vi "Parse Response JSON.vi"(8 "error in (no error)":errorcluster, 10 "Response JSON":string, 11 "RGetSceneList in":refnum<class "RGetSceneList.lvclass">) -> (0 "error out":errorcluster, 3 "RGetSceneList out":refnum<class "RGetSceneList.lvclass">)   [LabVIEW 2022 SP3, in "obs-websocket-lv.lvlib" / "RGetSceneList.lvclass"]
uses:
  RGetSceneList.lvclass
  RGetSceneList.lvclass/RGetSceneList.ctl
  <vilib>/IlluminatedG/lv-web-crypto/lv-json/JSON/JSON.lvlib
  Scene.ctl
  obs-websocket-lv.lvlib
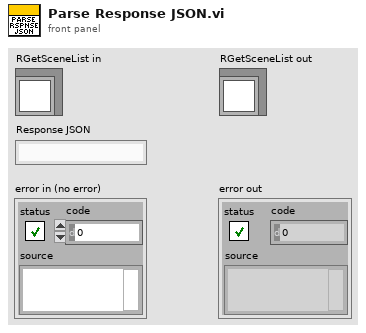
[diagram p1: front panel]
types:
  T1 = typedef "JSON.lvlib/JSON Item Type.ctl" = enum16{"unknown", "null", "Array", "Object", "String", "Number", "Boolean"}
  T2 = typedef "obs-websocket-lv.lvlib/Scene.ctl" = cluster{"Index":i32, "Name":string}
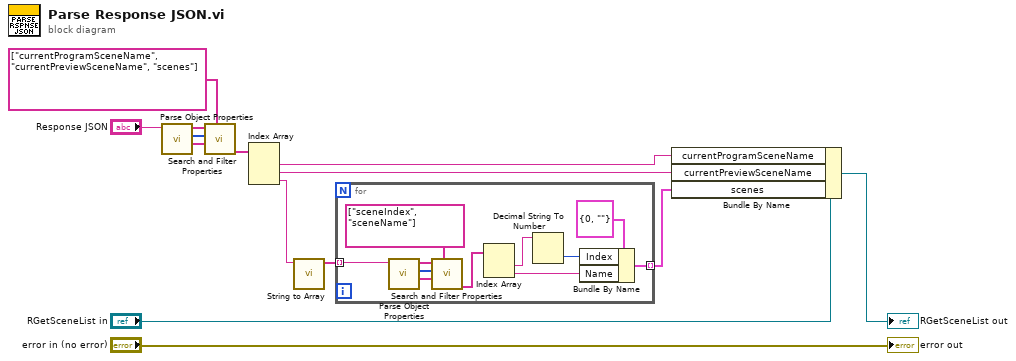
[diagram p0: block diagram]
diagram:
  n1 = call <vilib>:"Parse Object Properties.vi"("JSON String"="Response JSON") -> ("Values"=w10:string[], "Item Types"=w11:T1[], "Keys"=w12:string[])  [unwired: 7 in, 1 out]
  n2 = call <vilib>:"Search and Filter Properties.vi"("Search Keys"=string[] ["currentProgramSceneName", "currentPreviewSceneName", "scenes"], "Values In"=w10, "Types In"=w11, "Keys In"=w12) -> ("Filtered Values"=w8:string[])  [unwired: 2 in, 5 out]
  n3 = Index Array(array=w8) -> (element #1=w7:string, element #2=w6:string, element #3=w5:string)  [unwired: 3 in]
  n4 = call <vilib>:"String to Array.vi"("Array String In"=w5) -> ("JSON Strings"=w4:string[])  [unwired: 10 in]
  n5 = for {
    tunnel: w4 -> [w23] mode=indexing
    tunnel: [w15] -> w3 mode=indexing
    n6 = call <vilib>:"Parse Object Properties.vi"("JSON String"=w23) -> ("Values"=w25:string[], "Item Types"=w24:T1[], "Keys"=w21:string[])  [unwired: 7 in, 1 out]
    n7 = call <vilib>:"Search and Filter Properties.vi"("Search Keys"=string[] ["sceneIndex", "sceneName"], "Values In"=w25, "Types In"=w24, "Keys In"=w21) -> ("Filtered Values"=w20:string[])  [unwired: 2 in, 5 out]
    n8 = Index Array(array=w20) -> (element #1=w19:string, element #2=w17:string)  [unwired: 2 in]
    n9 = Decimal String To Number(string=w19) -> (number=w16:i32)  [unwired: 2 in, 1 out]
    n10 = Bundle By Name(cluster=T2 {"Index"=0, "Name"=""} ("Scene"), "Index"=w16, "Name"=w17) -> (w15:T2)
  }
  n11 = Bundle By Name(cluster="RGetSceneList in", "currentProgramSceneName"=w7, "currentPreviewSceneName"=w6, "scenes"=w3) -> (→"RGetSceneList out":refnum<class "RGetSceneList.lvclass">)
  "error out" <- "error in (no error)"
